vi "Query Current Max.vi"(8 "error in (no error)":errorcluster, 11 "VISA resource name":refnum<visa-resource-name>) -> (0 "error out":errorcluster, 2 "Current Max (A)":dbl format="%.2f", 3 "VISA resource name out":refnum<visa-resource-name>)   [LabVIEW 2021, in "Sorensen M9A Series.lvlib"]
doc: "This VI returns the value of the soft current limit. Units are Amps."
uses:
  Sorensen M9A Series.lvlib
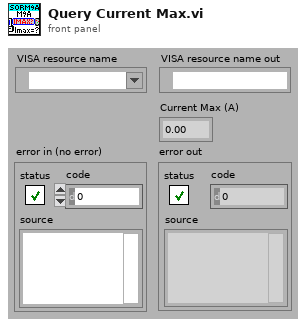
[diagram p1: front panel]
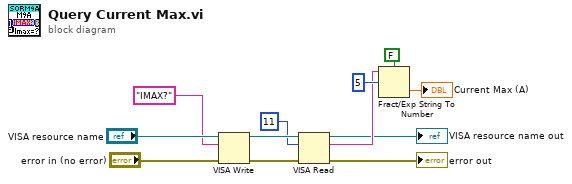
[diagram p0: block diagram]
diagram:
  n1 = VISA Write(VISA resource name="VISA resource name", write buffer="IMAX?" ("data"), error in (no error)="error in (no error)") -> (VISA resource name out=w7:refnum<visa-resource-name>, error out=w6:errorcluster)  [unwired: 1 out]
  n2 = VISA Read(VISA resource name=w7, byte count=11, error in (no error)=w6) -> (VISA resource name out=→"VISA resource name out":refnum<visa-resource-name>, read buffer=w4:string, error out=→"error out":errorcluster)  [unwired: 1 out]
  n3 = Fract/Exp String To Number(use system decimal point (T)=FALSE, string=w4, offset=5) -> (number=→"Current Max (A)":dbl)  [unwired: 1 in, 1 out]
